vi "Control loop type mMc.vi"(0 "Loop in":i8(slide) caption="Control loop in" min=0 max=3 scale=0.0..3.0, 1 "Port":T1={"P type"=0, "reference"="", " Terminator "="\r\n", "Timeout"=300} {"Timeout" step=10; "P type" items=["none", "RS-232C"]}, 3 "error in (no error)":errorcluster, 4 "set/get":bool caption="set\n\n\nget", 5 "Controller #":string) -> (6 "Loop out":i8(slide) caption="Control loop out" scale=0.0..3.0, 9 "error out":errorcluster)   [LabVIEW 2013]
panel:
  # "Control loop type"
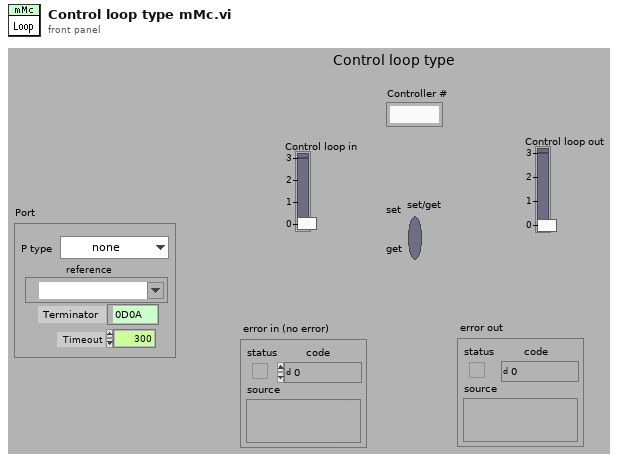
[diagram p1: front panel]
types:
  T1 = cluster{"P type":u16, "reference":refnum<visa-resource-name>, " Terminator ":string, "Timeout":i32}
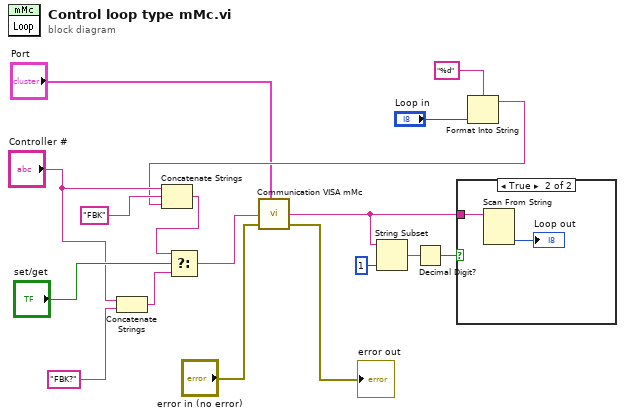
[diagram p0: block diagram]
diagram:
  n1 = Concatenate Strings("Controller #", "FBK?") -> (w17:string)
  n2 = Format Into String(format string="%d", "Loop in") -> (resulting string=w7:string)  [unwired: 2 in, 1 out]
  n3 = Concatenate Strings("Controller #", "FBK", w7) -> (w15:string)
  n4 = Select(t=w15, s="set/get", f=w17) -> (s? t:f=w14:string)
  n5 = call "Communication VISA mMc.vi"("Port"="Port", "Command"=w14, "error in (no error)"="error in (no error)") -> ("Return"=w1:string, "error out"=→"error out":errorcluster)  [unwired: 3 in, 2 out]
  n6 = String Subset(string=w1, length (rest)=1 ("length (rest)")) -> (substring=w3:string)  [unwired: 1 in]
  n7 = Decimal Digit?(1:w3) -> (0:w2:bool)
  n8 = case shown="True" w2 {
    tunnel: w1 -> [_ w19]
    frame False {
    }
    frame True {
      n9 = Scan From String(input string=w19) -> (output 1=→"Loop out":i8)  [unwired: 4 in, 3 out]
    }
  }
